vi "Archivo_v2.vi"(5 "Error In":errorcluster) -> (14 "selected path":path, 15 "cancelled":bool, 19 "Error Out":errorcluster)   [LabVIEW 2013]
doc: "Se guardan las imagenes en formato *.TIF o *.PNG para que puedan ser procesadas.\nSe hace la conversion de *.DAT a uno de estos dos formatos, se debe indicar en donde estan ubicados los archivos *.DAT y en donde queremos guardar las imagenes ya convertidas."
uses:
  <vilib>/Utility/sysdir.llb/System Directory Type.ctl
  <vilib>/ErrorRing/Error Ring.xnode
panel:
  out "exists":bool
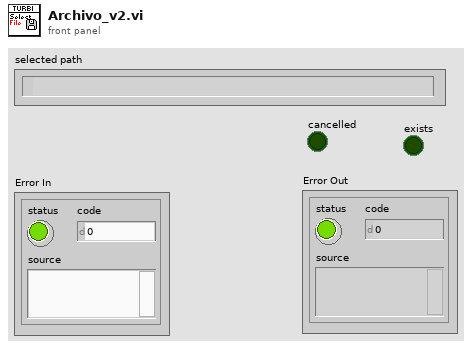
[diagram p1: front panel]
types:
  T1 = enum16{"open", "replace", "create", "open or create", "replace or create", "replace or create with confirmation"}
  T2 = typedef "System Directory Type.ctl" = i32
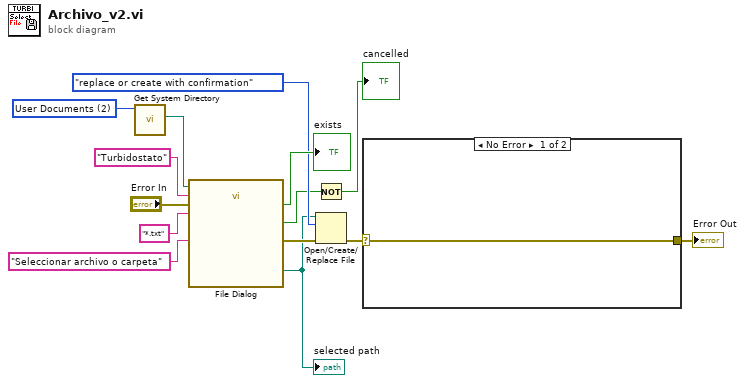
[diagram p0: block diagram]
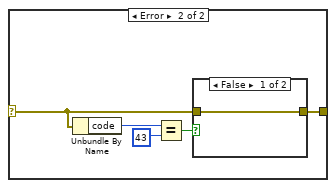
[diagram p2: hidden frame]
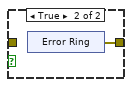
[diagram p3: hidden frame]
diagram:
  w13 = T2 2 items=["User Home"=0, "User Desktop"=1, "User Documents"=2, "User Application Data"=3, "User Preferences"=4, "User Temporary"=5, "Public Documents"=6, "Public Application Data"=7, "Public Preferences"=8, "Public Cache"=13, "System Core Libraries"=9, "System Installed Libraries"=10, "Application Files"=11, "Boot Volume Root"=12] ("system directory type")
  n1 = call <vilib>:"Get System Directory.vi"("system directory type"=w13) -> ("system directory"=w14:path)  [unwired: 10 in]
  n2 = call "File Dialog"("start path"=w14, "prompt"="Seleccionar archivo o carpeta", "default name"="Turbidostato", "error in"="Error In", "pattern (all files)"="*.txt") -> ("selected path"=w3:path, "exists"=→"exists":bool, "cancelled"=w5:bool, "error out"=w8:errorcluster)  [unwired: 7 in]
  "selected path" <- w3
  n3 = Not(x=w5) -> (.not. x?=→"cancelled":bool)
  n4 = Open/Create/Replace File(file path (use dialog)=w3, error in=w8, operation (0:open)=T1."replace or create with confirmation") -> (error out=w2:errorcluster)  [unwired: 3 in, 2 out]
  n5 = case shown="No Error" w2 {
    selector: w2 -> [w15 w16]
    tunnel: [w15 w17] -> w1
    frame No Error {
    }
    frame Error {
      n6 = Unbundle By Name(w16) -> ("code"=w20:i32)
      n7 = Equal?(x=w20, y=43) -> (x = y?=w18:bool)
      n8 = case shown="False" w18 {
        tunnel: [w21 w22] -> w17
        tunnel: w16 -> [w21 _]
        frame False {
        }
        frame True {
          n9 = xnode "Error Ring"() -> ("error out"=w22:errorcluster)
        }
      }
    }
  }
  "Error Out" <- w1
